vi "Main.vi"() -> ()   [LabVIEW 2018]
uses:
  Initialize/CreateQueue/AllDataQueue.ctl
  Initialize/CreateQueue/SocketQueue.ctl
  Initialize/CreateQueue/LogDataQueue.ctl
  Initialize/CreateQueue/ProDataQueue.ctl
  ProData/SettingData.ctl
  socket/socket.ctl
  Initialize/Setting/DA.ctl
  Initialize/Setting/AD.ctl
  ProData/prodatascan.ctl
  Support/Data.ctl
  <vilib>/DAQmx/read.llb/DAQmx Read (Analog Wfm 1Chan NSamp).vi
  <vilib>/DAQmx/write.llb/DAQmx Write (Analog DBL 1Chan 1Samp).vi
  <vilib>/DAQmx/create/channels.llb/DAQmx Create Channel (AI-Voltage-Basic).vi
  <vilib>/DAQmx/configure/timing.llb/DAQmx Timing (Sample Clock).vi
  <vilib>/DAQmx/miscellaneous.llb/DAQmx Fill In Error Info.vi
  <vilib>/DAQmx/create/channels.llb/DAQmx Create Channel (AO-Voltage-Basic).vi
panel:
  in  "选项卡控件":enum32{"Setting", "Chart"}(tab)
  in  "端口":u16=10020
  in  "timeout":i16=-1
  in  "标准差倍数":dbl=7.0
  in  "normal":string="1"
  in  "每通道采样率":u16=60
  in  "电压最大值":u16=5
  in  "电压最小值":i16=-5
  in  "采样率":u16=60000
  in  "接线方式":i32(ring)=10106 items=["默认"=-1, "RSE"=10083, "NRSE"=10078, "差分"=10106, "伪差分"=12529]
  in  "采样模式":i32(ring)=10123 items=["有限采样"=10178, "连续采样"=10123, "硬件定时单点"=12522]
  in  "DA电压最大值":dbl=10.0
  in  "DA电压最小值":dbl=-10.0
  in  "选择通道AD":tag="USB_6211_2/ai1"
  in  "选择通道DA":tag="USB_6211_2/ao1"
  in  "地址":string="8.131.237.84"
  out "选择通道AD  2":tag="USB_6211_2/ai1"
  out "连接状态":string="连接成功"
  in  "adjust":dbl=0.1
  out "波形图表":i32(graph)
  out "nvpai":dbl
  out "max":dbl
  out "min":dbl
  in  "等待时间（毫秒）":u32=15
  out "ADchart":dbl(graph)
  out "DAchart":dbl(graph)
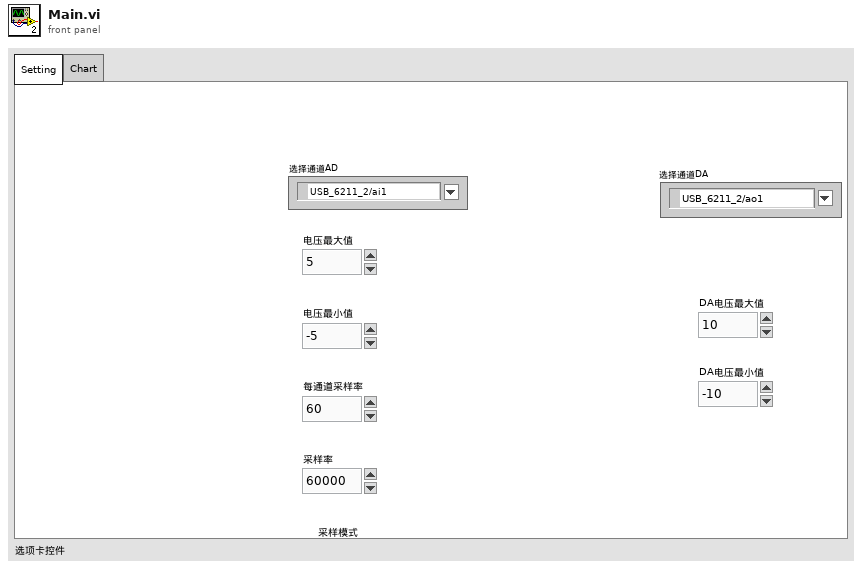
[diagram p1: front panel]
types:
  T1 = typedef "socket.ctl" = cluster{"端口":u16, "timeout":u16, "标准差倍数":dbl, "address":string, "abnormal":string}
  T2 = typedef "DA.ctl" = cluster{"电压最大值":dbl, " 电压最小值":dbl, "选择通道DA ":tag}
  T3 = typedef "AD.ctl" = cluster{"电压最大值":u16, " 电压最小值":i16, " 采样率":u16, "每通道采样率":u16, "采样模式":i32, "接线方式":i32, "source":tag, "选择通道AD ":tag}
  T4 = typedef "Data.ctl" = cluster{"SynQueue":cluster{"SocketQueue":T5, "LogQueue":T6, " DA":refnum<queue>, "ProQueue":T7}, "Error":cluster{"错误输出 2":errorcluster}, "SettingData":T8}
  T5 = typedef "SocketQueue.ctl" = cluster{"ADSTDqueue ":refnum<queue>, "SocketADExceptionqueue":refnum<queue>, "  SocketAD":refnum<queue>}
  T6 = typedef "LogDataQueue.ctl" = cluster{"RunningADqueue":refnum<queue>, "Compensatequeue":refnum<queue>, " RunningDAqueue":refnum<queue>, " RunMin":refnum<queue>}
  T7 = typedef "ProDataQueue.ctl" = cluster{"buffer ":refnum<queue>, " StimeADqueue":refnum<queue>, "  MtimeADqueue":refnum<queue>}
  T8 = typedef "SettingData.ctl" = cluster{"socket":T1, "DA":T2, "AD":T3, "prodatascan":T9}
  T9 = typedef "prodatascan.ctl" = cluster{"max":dbl, "min":dbl, " nvpai":dbl, "初始化数组":dbl[]}
  T10 = typedef "AllDataQueue.ctl" = cluster{"SocketQueue":T5, "LogQueue":T6, " DA":refnum<queue>, "ProQueue":T7}
  T11 = cluster{"max":dbl, "min":dbl, " nvpai":dbl, "初始化数组":dbl[]}
  T12 = cluster{"SocketQueue":T5, "LogQueue":T6, " DA":refnum<queue>, "ProQueue":T7}
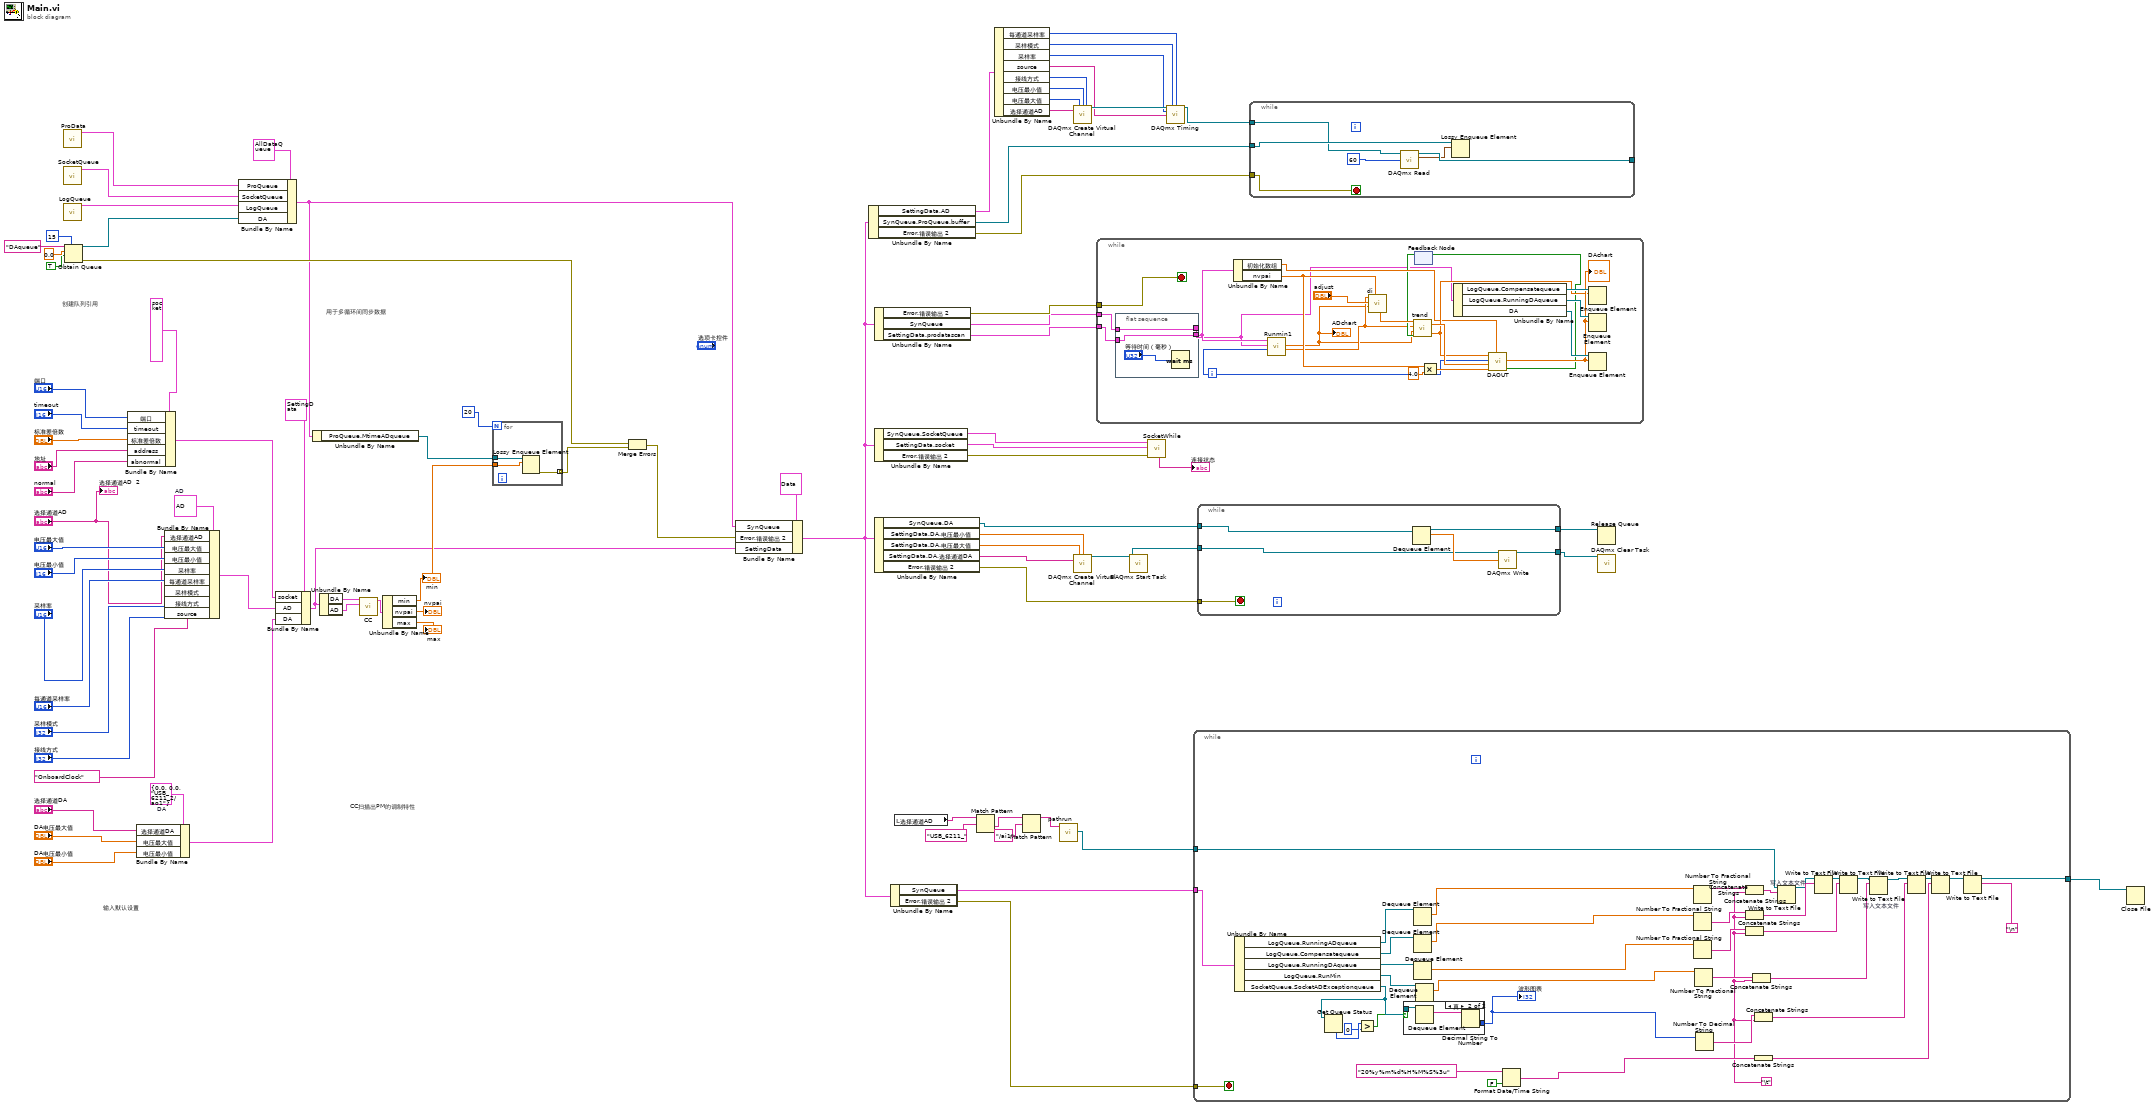
[diagram p0: block diagram]
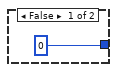
[diagram p2: hidden frame]
diagram:
  w8 = T2 {"电压最大值"=0.0, " 电压最小值"=0.0, "选择通道DA "="USB_6211_2/ao1"}  # DA
  w9 = T3 {"电压最大值"=10013, " 电压最小值"=10013, " 采样率"=10013, "每通道采样率"=10013, "采样模式"=10123, "接线方式"=10106, "source"="OnboardClock", "选择通道AD "="USB_6211_2/ai1"}  # AD
  # "CC扫描出PM的调制特性"
  # "输入默认设置"
  # "用于多循环间同步数据"
  # "创建队列引用"
  n1 = call "ProData.vi"() -> ("ProDataQueue"=w77:T7)  [unwired: 11 in]
  n2 = call "SocketQueue.vi"() -> ("SocketQueue"=w79:T5)  [unwired: 11 in]
  n3 = call "LogQueue.vi"() -> ("LogQueue"=w78:T6)  [unwired: 11 in]
  n4 = Obtain Queue(max queue size (-1, unlimited)=15 ("队列最大值（-1，无限）"), name (unnamed)="DAqueue" ("名称（未命名）"), element data type=0.0, create if not found? (T)=TRUE ("如未找到则创建？(T)")) -> (queue out=w80:refnum<queue>, error out=w52:errorcluster)  [unwired: 1 in, 1 out]
  n5 = Bundle By Name(cluster=T1 {"端口"=10013, "timeout"=10013, "标准差倍数"=0.0, "address"="{\"ad\":1}", "abnormal"="{\"ad\":0}"} ("socket"), "端口"="端口", "timeout"="timeout", "标准差倍数"="标准差倍数", "address"="地址", "abnormal"="normal") -> (w65:T1)
  n6 = Bundle By Name(cluster=w8, "选择通道DA"="选择通道DA", "电压最大值"="DA电压最大值", "电压最小值"="DA电压最小值") -> (w60:T2)
  n7 = Bundle By Name(cluster=w9, "选择通道AD"="选择通道AD", "电压最大值"="电压最大值", "电压最小值"="电压最小值", "采样率"="采样率", "每通道采样率"="每通道采样率", "采样模式"="采样模式", "接线方式"="接线方式", "source"=tag "OnboardClock") -> (w58:T3)
  n8 = Bundle By Name(cluster=T10 {"SocketQueue"={"ADSTDqueue "=refnum, "SocketADExceptionqueue"=refnum, "  SocketAD"=refnum}, "LogQueue"={"RunningADqueue"=refnum, "Compensatequeue"=refnum, " RunningDAqueue"=refnum, " RunMin"=refnum}, " DA"=refnum, "ProQueue"={"buffer "=refnum, " StimeADqueue"=refnum, "  MtimeADqueue"=refnum}}, "ProQueue"=w77, "SocketQueue"=w79, "LogQueue"=w78, "DA"=w80) -> (w40:T10)
  n9 = Bundle By Name(cluster=T8 {"socket"={"端口"=10013, "timeout"=10013, "标准差倍数"=0.0, "address"="{\"ad\":1}", "abnormal"="{\"ad\":0}"}, "DA"={"电压最大值"=0.0, " 电压最小值"=0.0, "选择通道DA "="USB_6211_2/ao1"}, "AD"={"电压最大值"=10013, " 电压最小值"=10013, " 采样率"=10013, "每通道采样率"=10013, "采样模式"=10123, "接线方式"=10106, "source"="OnboardClock", "选择通道AD "="USB_6211_2/ai1"}, "prodatascan"={"max"=0.0, "min"=0.0, " nvpai"=0.0, "初始化数组"=[]}} ("SettingData"), "socket"=w65, "AD"=w58, "DA"=w60) -> (w46:T8)
  n10 = Unbundle By Name(w40) -> ("ProQueue.MtimeADqueue"=w54:refnum<queue>)
  n11 = Unbundle By Name(w46) -> ("DA"=w56:T2, "AD"=w57:T3)
  n12 = call "CC.vi"("AD"=w57, "DA"=w56) -> ("prodatascan"=w47:T11)  [unwired: 8 in, 1 out]
  n13 = Unbundle By Name(w47) -> ("min"=w55:dbl, "nvpai"=→"nvpai":dbl, "max"=→"max":dbl)
  "min" <- w55
  n14 = for {
    N: 20 -> [_]
    tunnel: w54 -> [w88]
    tunnel: w55 -> [w87]
    tunnel: [w86] -> w51 mode=indexing
    n15 = Lossy Enqueue Element(queue=w88, element=w87) -> (error out=w86:errorcluster)  [unwired: 1 in, 3 out]
  }
  n16 = Merge Errors(w52, w51) -> (w30:errorcluster)
  n17 = Bundle By Name(cluster=T4 {"SynQueue"={"SocketQueue"={"ADSTDqueue "=refnum, "SocketADExceptionqueue"=refnum, "  SocketAD"=refnum}, "LogQueue"={"RunningADqueue"=refnum, "Compensatequeue"=refnum, " RunningDAqueue"=refnum, " RunMin"=refnum}, " DA"=refnum, "ProQueue"={"buffer "=refnum, " StimeADqueue"=refnum, "  MtimeADqueue"=refnum}}, "Error"={"错误输出 2"={"status"=FALSE, "code"=0, "source"=""}}, "SettingData"={"socket"={"端口"=0, "timeout"=0, "标准差倍数"=0.0, "address"="{\"ad\":1}", "abnormal"="{\"ad\":0}"}, "DA"={"电压最大值"=0.0, " 电压最小值"=0.0, "选择通道DA "="USB_6211_2/ao1"}, "AD"={"电压最大值"=10013, " 电压最小值"=10013, " 采样率"=10013, "每通道采样率"=10013, "采样模式"=10123, "接线方式"=10106, "source"="OnboardClock", "选择通道AD "="USB_6211_2/ai1"}, "prodatascan"={"max"=0.0, "min"=0.0, " nvpai"=0.0, "初始化数组"=[]}}}, "SynQueue"=w40, "Error.错误输出 2"=w30, "SettingData"=w46) -> (w15:T4)
  n18 = Unbundle By Name(w15) -> ("SettingData.AD"=w18:T3, "SynQueue.ProQueue.buffer"=w28:refnum<queue>, "Error.错误输出 2"=w29:errorcluster)
  n19 = Unbundle By Name(w15) -> ("Error.错误输出 2"=w43:errorcluster, "SynQueue"=w41:T12, "SettingData.prodatascan"=w42:T9)
  n20 = Unbundle By Name(w15) -> ("SynQueue.SocketQueue"=w44:T5, "SettingData.socket"=w2:T1, "Error.错误输出 2"=w45:errorcluster)
  n21 = Unbundle By Name(w15) -> ("SynQueue.DA"=w34:refnum<queue>, "SettingData.DA.电压最小值"=w37:dbl, "SettingData.DA.电压最大值"=w33:dbl, "SettingData.DA.选择通道DA"=w38:tag, "Error.错误输出 2"=w39:errorcluster)
  n22 = Unbundle By Name(w15) -> ("SynQueue"=w14:T12, "Error.错误输出 2"=w13:errorcluster)
  n23 = local read "选择通道AD"() -> (w7:tag)
  n24 = Match Pattern(string=w7, regular expression="USB_6211_" ("正则表达式")) -> (after substring=w5:string)  [unwired: 1 in, 3 out]
  n25 = Unbundle By Name(w18) -> ("每通道采样率"=w19:u16, "采样模式"=w20:i32, "采样率"=w21:u16, "source"=w22:tag, "接线方式"=w27:i32, "电压最小值"=w26:i16, "电压最大值"=w25:u16, "选择通道AD"=w24:tag)
  n26 = Match Pattern(string=w5, regular expression="/ai1" ("正则表达式")) -> (before substring=w3:string)  [unwired: 1 in, 3 out]
  n27 = call "pathrun.vi"("时间格式字符串(%c)"=w3) -> ("引用句柄输出"=w16:refnum<file>)  [unwired: 10 in]
  n28 = call-poly <vilib>:"DAQmx Create Virtual Channel.vi"("maximum value"=w25, "minimum value"=w26, "input terminal configuration"=w27, "physical channels"=w24) -> ("task out"=w23:refnum<k21>)  [unwired: 10 in, 1 out]
  n29 = call-poly <vilib>:"DAQmx Create Virtual Channel.vi"("maximum value"=w33, "minimum value"=w37, "physical channels"=w38) -> ("task out"=w36:refnum<k21>)  [unwired: 11 in, 1 out]
  n30 = while {
    tunnel: w43 -> [w108]
    tunnel: w41 -> [w90]
    tunnel: w42 -> [w92]
    i -> [w96]
    stop <- w108 stop-if-true
    n31 = flat-sequence {
      tunnel: w92 -> [w112]
      tunnel: [w112] -> w91
      tunnel: w90 -> [w111]
      tunnel: [w111] -> w89
      frame #0 {
        n32 = Wait (ms)(milliseconds to wait="等待时间（毫秒）") -> ()  [unwired: 1 out]
      }
    }
    n33 = Unbundle By Name(w91) -> ("初始化数组"=w99:dbl[], "nvpai"=w95:dbl)
    n34 = call "Runmin1.vi"("循环次数 i"=w96, "Queue1"=w89, "prodatascan"=w91) -> ("runMin"=w94:dbl, "AD"=w93:dbl)  [unwired: 7 in]
    "ADchart" <- w93
    n35 = call "di.vi"("RunMin"=w94, "adjust"="adjust", "AD"=w93, "Nvpai"=w95) -> ("Compensate1"=w109:dbl)  [unwired: 6 in]
    n36 = feedback #1() -> (w97:bool)  [unwired: 1 in]
    n37 = call "trend.vi"("jumpBool"=w97, "AD"=w93, "runMin"=w94, "Compensate1"=w109) -> ("Compensate1Out"=w100:dbl, "changeSymbol"=w101:dbl)
    n38 = Multiply(x=w95, y=4.0) -> (x*y=w102:dbl)
    n39 = Unbundle By Name(w89) -> ("LogQueue.Compensatequeue"=w107:refnum<queue>, "LogQueue.RunningDAqueue"=w106:refnum<queue>, "DA"=w104:refnum<queue>)
    n40 = call "DAOUT.vi"("maxInitial数组"=w99, "maxInitialVoltage"=w102, "changeSymbol"=w101, "running recycle counter"=w96, "compensate"=w100) -> ("jump symbol"=w98:bool, "real running DA output"=w103:dbl)  [unwired: 5 in]
    "DAchart" <- w103
    n41 = feedback-in #1(w98) -> ()
    n42 = Enqueue Element(queue=w107, element=w100) -> ()  [unwired: 2 in, 3 out]
    n43 = Enqueue Element(queue=w106, element=w103) -> ()  [unwired: 2 in, 3 out]
    n44 = Enqueue Element(queue=w104, element=w103) -> ()  [unwired: 2 in, 3 out]
  }
  n45 = call <vilib>:"DAQmx Start Task.vi"("task/channels in"=w36) -> ("task out"=w35:refnum<k21>)  [unwired: 13 in, 1 out]
  n46 = call "SocketWhile.vi"("error out"=w45, "socket 2"=w2, "SocketQueue"=w44) -> ("socket"=→"连接状态":string)  [unwired: 8 in]
  n47 = call-poly <vilib>:"DAQmx Timing.vi"("task/channels in"=w23, "sample mode"=w20, "samples per channel"=w19, "rate"=w21, "source"=w22) -> ("task out"=w17:refnum<k21>)  [unwired: 9 in, 1 out]
  n48 = while {
    tunnel: w13 -> [w147]
    tunnel: [w117] -> w12
    tunnel: w16 -> [w116]
    tunnel: w14 -> [w114]
    stop <- w147 stop-if-true
    w115 = "\t"
    n49 = Unbundle By Name(w114) -> ("LogQueue.RunningADqueue"=w146:refnum<queue>, "LogQueue.Compensatequeue"=w150:refnum<queue>, "LogQueue.RunningDAqueue"=w149:refnum<queue>, "LogQueue.RunMin"=w148:refnum<queue>, "SocketQueue.SocketADExceptionqueue"=w145:refnum<queue>)
    n50 = Get Queue Status(queue=w145) -> (# elements in queue=w144:i32)  [unwired: 2 in, 7 out]
    n51 = Greater?(x=w144, y=0) -> (0:w142:bool)
    n52 = case shown="真" w142 {
      tunnel: [0 w155] -> w122
      tunnel: w145 -> [_ w154]
      frame False {
      }
      frame True {
        n53 = Dequeue Element(queue=w154) -> (element=w156:string)  [unwired: 2 in, 3 out]
        n54 = Decimal String To Number(string=w156) -> (number=w155:i32)  [unwired: 2 in, 1 out]
      }
    }
    "波形图表" <- w122
    n55 = Dequeue Element(queue=w146) -> (element=w132:dbl)  [unwired: 2 in, 3 out]
    n56 = Dequeue Element(queue=w150) -> (element=w131:dbl)  [unwired: 2 in, 3 out]
    n57 = Dequeue Element(queue=w149) -> (element=w130:dbl)  [unwired: 2 in, 3 out]
    n58 = Dequeue Element(queue=w148) -> (element=w124:dbl)  [unwired: 2 in, 3 out]
    n59 = Format Date/Time String(time format string (%c)="20%y%m%d%H%M%S%3u" ("时间格式字符串(%c)"), UTC format=FALSE ("UTC格式")) -> (date/time string=w120:string)  [unwired: 1 in]
    n60 = Number To Fractional String(number=w132) -> (F-format string=w137:string)  [unwired: 3 in]
    n61 = Number To Fractional String(number=w131) -> (F-format string=w139:string)  [unwired: 3 in]
    n62 = Number To Fractional String(number=w130) -> (F-format string=w140:string)  [unwired: 3 in]
    n63 = Number To Fractional String(number=w124) -> (F-format string=w125:string)  [unwired: 3 in]
    n64 = Number To Decimal String(number=w122) -> (decimal integer string=w121:string)  [unwired: 1 in]
    n65 = Concatenate Strings(w137, w115) -> (w134:string)
    n66 = Concatenate Strings(w139, w115) -> (w136:string)
    n67 = Concatenate Strings(w140, w115) -> (w141:string)
    n68 = Concatenate Strings(w125, w115) -> (w123:string)
    n69 = Concatenate Strings(w121, w115) -> (w119:string)
    n70 = Concatenate Strings(w120) -> (w118:string)
    n71 = Write to Text File "写入文本文件"(file (use dialog)=w116, text=w134) -> (refnum out=w135:refnum<file>)  [unwired: 2 in, 2 out]
    n72 = Write to Text File(file (use dialog)=w135, text=w136) -> (refnum out=w138:refnum<file>)  [unwired: 2 in, 2 out]
    n73 = Write to Text File(file (use dialog)=w138, text=w141) -> (refnum out=w127:refnum<file>)  [unwired: 2 in, 2 out]
    n74 = Write to Text File "写入文本文件"(file (use dialog)=w127, text=w123) -> (refnum out=w128:refnum<file>)  [unwired: 2 in, 2 out]
    n75 = Write to Text File(file (use dialog)=w128, text=w119) -> (refnum out=w129:refnum<file>)  [unwired: 2 in, 2 out]
    n76 = Write to Text File(file (use dialog)=w129, text=w118) -> (refnum out=w126:refnum<file>)  [unwired: 2 in, 2 out]
    n77 = Write to Text File(file (use dialog)=w126, text="\n") -> (refnum out=w117:refnum<file>)  [unwired: 2 in, 2 out]
  }
  n78 = while {
    tunnel: [w162] -> w31
    tunnel: [w161] -> w32
    tunnel: w34 -> [w158]
    tunnel: w39 -> [w159]
    tunnel: w35 -> [w157]
    stop <- w159 stop-if-true
    n79 = Dequeue Element(queue=w158) -> (queue out=w161:refnum<queue>, element=w160:dbl)  [unwired: 2 in, 2 out]
    n80 = call-poly <vilib>:"DAQmx Write.vi"("task/channels in"=w157, "data"=w160) -> ("task out"=w162:refnum<k21>)  [unwired: 11 in, 2 out]
  }
  n81 = while {
    tunnel: [w168] -> _
    tunnel: w28 -> [w165]
    tunnel: w29 -> [w164]
    tunnel: w17 -> [w163]
    stop <- w164 stop-if-true
    n82 = call-poly <vilib>:"DAQmx Read.vi"("task/channels in"=w163, "number of samples per channel"=60) -> ("task out"=w168:refnum<k21>, "data"=w167:waveform(dbl))  [unwired: 11 in, 1 out]
    n83 = Lossy Enqueue Element(queue=w165, element=w167) -> ()  [unwired: 1 in, 4 out]
  }
  n84 = Release Queue(queue=w32) -> ()  [unwired: 2 in, 3 out]
  n85 = call <vilib>:"DAQmx Clear Task.vi"("task in"=w31) -> ()  [unwired: 14 in, 1 out]
  n86 = Close File(refnum=w12) -> ()  [unwired: 1 in, 2 out]
  "选择通道AD  2" <- "选择通道AD"
